vi "SPIM_Record.vi"() -> ()   [LabVIEW 2012]
panel:
  out "XY Graph 2":cluster{"Y":dbl[], "Y":dbl[]}[](graph)
  out "XY Graph":cluster{"Y":dbl[], "Y":dbl[]}[](graph)
  out "Frames Recorded":i32
  in  "DCIMG Path":path
  in  "Frames":i32=100
  out "Error Out":errorcluster
  # "This is an example of how to use the\nhard disk recorder functions to record\nimages to a DCIMG file."
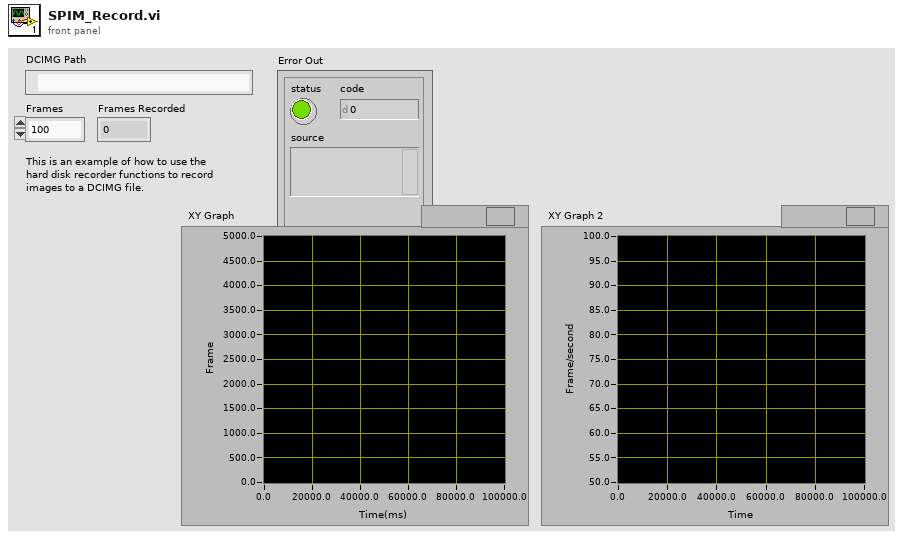
[diagram p1: front panel]
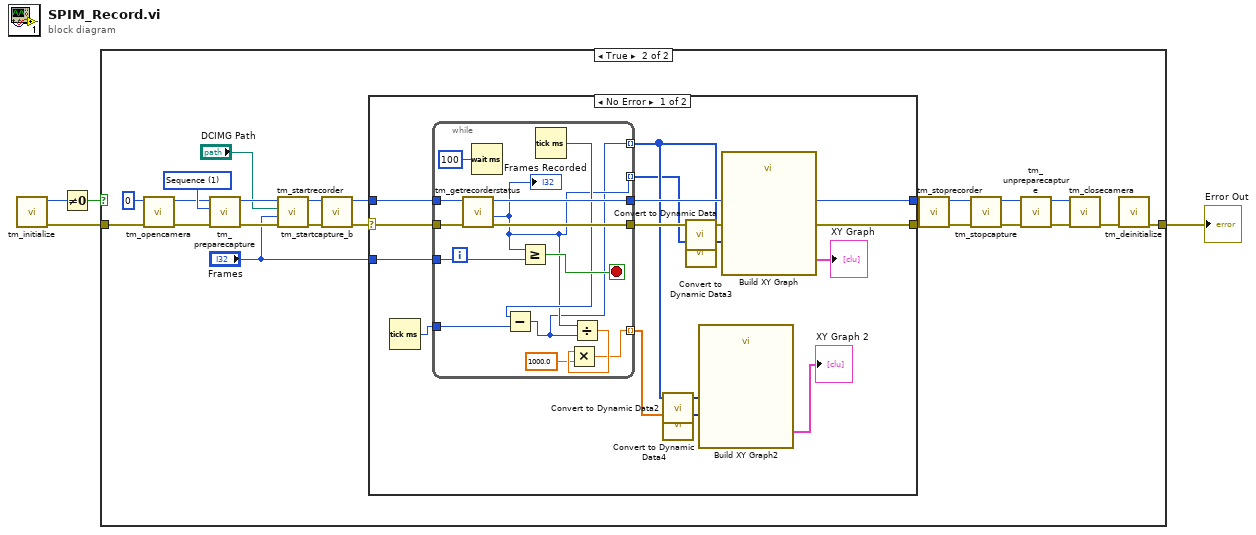
[diagram p0: block diagram]
diagram:
  n1 = call <userlib>:"tm_initialize.vi"() -> ("error out"=w1:errorcluster, "Number Of Cameras"=w2:u32)  [unwired: 10 in]
  n2 = Not Equal To 0?(x=w2) -> (x != 0?=w4:bool)
  n3 = case shown="True" w4 {
    tunnel: w1 -> [w5 w28]
    tunnel: [w5 w24] -> w3
    frame False {
    }
    frame True {
      w26 = 1 items=["Snap", "Sequence"] ("Capture mode")
      n4 = call <userlib>:"tm_opencamera.vi"("error in (no error)"=w28, "Camera Index"=u32 0) -> ("error out"=w12:errorcluster, "Handle out"=w13:u32)  [unwired: 8 in]
      n5 = call <userlib>:"tm_preparecapture.vi"("error in (no error)"=w12, "Capture mode"=w26, "Handle in"=w13) -> ("error out"=w21:errorcluster, "Handle out"=w20:u32)  [unwired: 5 in, 2 out]
      n6 = call <userlib>:"tm_startrecorder.vi"("error in (no error)"=w21, "frames"="Frames", "File"="DCIMG Path", "Handle in"=w20) -> ("error out"=w19:errorcluster, "Handle out"=w18:u32)  [unwired: 6 in]
      n7 = call <userlib>:"tm_startcapture_b.vi"("error in (no error)"=w19, "Handle in"=w18) -> ("error out"=w17:errorcluster, "Handle out"=w16:u32)  [unwired: 8 in]
      n8 = case shown="No Error" w17 {
        selector: w17 -> [w43 w58]
        tunnel: w16 -> [w42 w59]
        tunnel: [w37 w59] -> w6
        tunnel: [w41 w58] -> w7
        tunnel: "Frames" -> [w40 _]
        frame No Error {
          n9 = Tick Count (ms)() -> (millisecond timer value=w29:u32)
          n10 = while {
            tunnel: w43 -> [w55]
            tunnel: w42 -> [w54]
            tunnel: [w53] -> w41
            tunnel: [w56] -> w37
            tunnel: w40 -> [w57]
            tunnel: [w48] -> w35 mode=indexing
            tunnel: [w49] -> w33 mode=indexing
            tunnel: [w44] -> w31 mode=indexing
            tunnel: w29 -> [w47]
            stop <- w52 stop-if-true
            n11 = call <userlib>:"tm_getrecorderstatus.vi"("error in (no error)"=w55, "Handle"=w54) -> ("error out"=w53:errorcluster, "Count"=w49:i32, "Handle"=w56:u32)  [unwired: 6 in, 1 out]
            "Frames Recorded" <- w49
            n12 = Wait (ms)(milliseconds to wait=u32 100) -> ()  [unwired: 1 out]
            n13 = Greater Or Equal?(x=w49, y=w57) -> (x >= y?=w52:bool)
            n14 = Tick Count (ms)() -> (millisecond timer value=w50:u32)
            n15 = Subtract(x=w50, y=w47) -> (x-y=w48:u32)
            n16 = Divide(x=w49, y=w48) -> (x/y=w46:dbl)
            n17 = Multiply(x=w46, y=1000.0) -> (x*y=w44:dbl)
          }
          n18 = call "Convert to Dynamic Data2"("Array"=w35) -> ("Dynamic Data Type"=w34:dynamicdata)  [unwired: 3 in]
          n19 = call "Convert to Dynamic Data4"("Array"=w31) -> ("Dynamic Data Type"=w30:dynamicdata)  [unwired: 3 in]
          n20 = call "Convert to Dynamic Data"("Array"=w35) -> ("Dynamic Data Type"=w36:dynamicdata)  [unwired: 3 in]
          n21 = call "Convert to Dynamic Data3"("Array"=w33) -> ("Dynamic Data Type"=w32:dynamicdata)  [unwired: 3 in]
          n22 = call "Build XY Graph2"("Y Input"=w30, "X Input"=w34) -> ("XY Graph"=→"XY Graph 2":cluster{"Y":dbl[], "Y":dbl[]}[])  [unwired: 3 in, 6 out]
          n23 = call "Build XY Graph"("Y Input"=w32, "X Input"=w36) -> ("XY Graph"=→"XY Graph":cluster{"Y":dbl[], "Y":dbl[]}[])  [unwired: 3 in, 6 out]
        }
        frame Error {
        }
      }
      n24 = call <userlib>:"tm_stoprecorder.vi"("error in (no error)"=w7, "Handle in"=w6) -> ("error out"=w8:errorcluster, "Handle out"=w9:u32)  [unwired: 8 in]
      n25 = call <userlib>:"tm_stopcapture.vi"("error in (no error)"=w8, "Handle in"=w9) -> ("error out"=w11:errorcluster, "Handle out"=w10:u32)  [unwired: 8 in]
      n26 = call <userlib>:"tm_unpreparecapture.vi"("error in (no error)"=w11, "Handle in"=w10) -> ("error out"=w23:errorcluster, "Handle out"=w22:u32)  [unwired: 8 in]
      n27 = call <userlib>:"tm_closecamera.vi"("error in (no error)"=w23, "Handle in"=w22) -> ("error out"=w25:errorcluster)  [unwired: 9 in]
      n28 = call <userlib>:"tm_deinitialize.vi"("error in (no error)"=w25) -> ("error out"=w24:errorcluster)  [unwired: 10 in]
    }
  }
  "Error Out" <- w3
